vi "DAQmx连接验证.vi"(8 "error in":errorcluster caption="错误输入", 10 "被测":tag caption="物理通道", 11 "参考":tag caption="物理通道") -> (0 "error out":errorcluster caption="错误输出")   [LabVIEW 2015]
uses:
  <vilib>/DAQmx/create/channels.llb/DAQmx Create Channel (AI-Voltage-Basic).vi
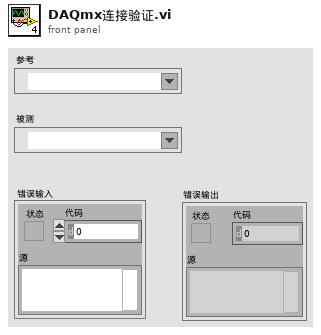
[diagram p1: front panel]
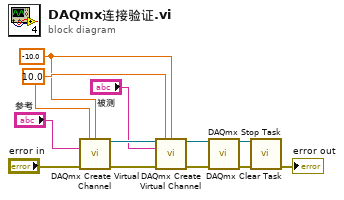
[diagram p0: block diagram]
diagram:
  w3 = -10.0 ("maximum value")
  w4 = 10.0 ("maximum value")
  n1 = call-poly <vilib>:"DAQmx Create Virtual Channel.vi"("maximum value"=w4, "minimum value"=w3, "physical channels"="参考", "error in"="error in") -> ("task out"=w7:refnum<k21>, "error out"=w2:errorcluster)  [unwired: 10 in]
  n2 = call-poly <vilib>:"DAQmx Create Virtual Channel.vi"("task in"=w7, "maximum value"=w4, "minimum value"=w3, "physical channels"="被测", "error in"=w2) -> ("task out"=w10:refnum<k21>, "error out"=w9:errorcluster)  [unwired: 9 in]
  n3 = call <vilib>:"DAQmx Stop Task.vi"("task/channels in"=w10, "error in"=w9) -> ("task out"=w12:refnum<k21>, "error out"=w11:errorcluster)  [unwired: 12 in]
  n4 = call <vilib>:"DAQmx Clear Task.vi"("task in"=w12, "error in"=w11) -> ("error out"=→"error out":errorcluster)  [unwired: 13 in]
